vi "write_data.vi"(8 "error in (no error)":errorcluster, 10 "data":T1, 11 "FeatureAgglomeration in":refnum<class "FeatureAgglomeration.lvclass">) -> (0 "error out":errorcluster, 3 "FeatureAgglomeration out":refnum<class "FeatureAgglomeration.lvclass">)   [LabVIEW 2020, in "FeatureAgglomeration.lvclass"]
uses:
  FeatureAgglomeration.lvclass
  Controls/feature_agglomeration_data.ctl
  FeatureAgglomeration.lvclass/FeatureAgglomeration.ctl
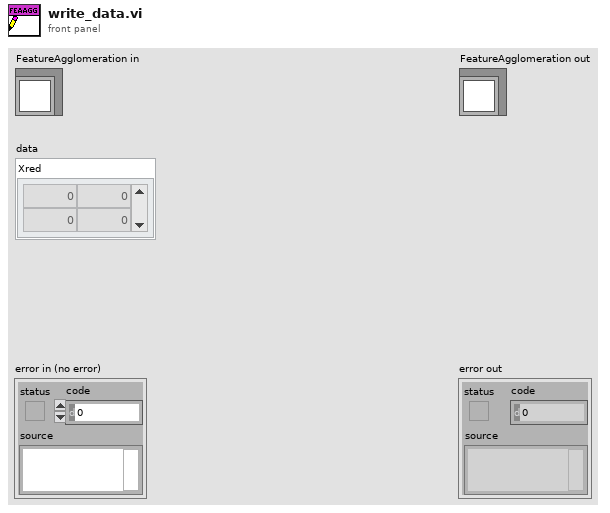
[diagram p1: front panel]
types:
  T1 = typedef "feature_agglomeration_data.ctl" = cluster{"Xred":dbl[][]}
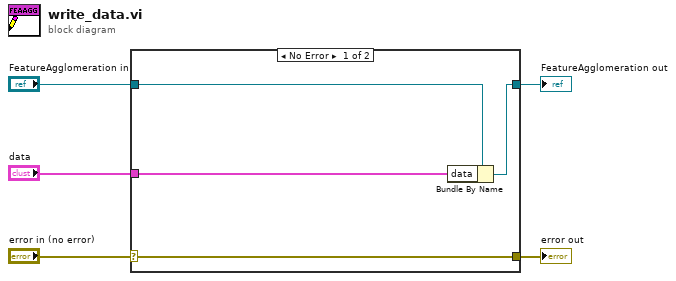
[diagram p0: block diagram]
diagram:
  n1 = case shown="No Error" "error in (no error)" {
    selector: "error in (no error)" -> [w9 w10]
    tunnel: [w9 w10] -> w4
    tunnel: [w7 w11] -> w2
    tunnel: "FeatureAgglomeration in" -> [w8 w11]
    tunnel: "data" -> [w6 _]
    frame No Error {
      n2 = Bundle By Name(cluster=w8, "data"=w6) -> (w7:refnum<class "FeatureAgglomeration.lvclass">)
    }
    frame Error {
    }
  }
  "error out" <- w4
  "FeatureAgglomeration out" <- w2
